vi "sign.vi"() -> ()   [LabVIEW 2020]
uses:
  <vilib>/Utility/file.llb/Read Delimited Spreadsheet (string).vi
  <vilib>/Utility/file.llb/Write Delimited Spreadsheet (string).vi
panel:
  out "output array":string[][](array[string])
  in  "请输入账号":string caption="Please enter your account:"
  in  "请输入密码":string caption="Please enter your password:"
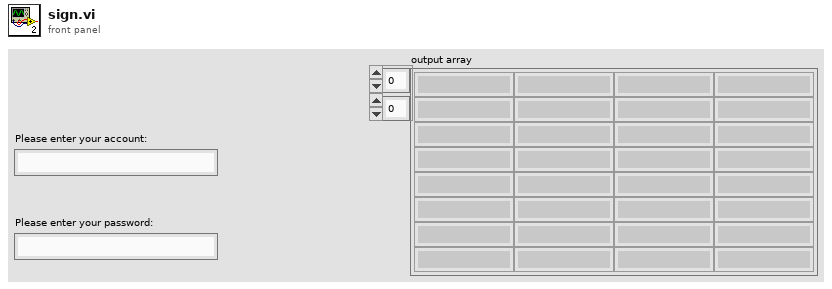
[diagram p1: front panel]
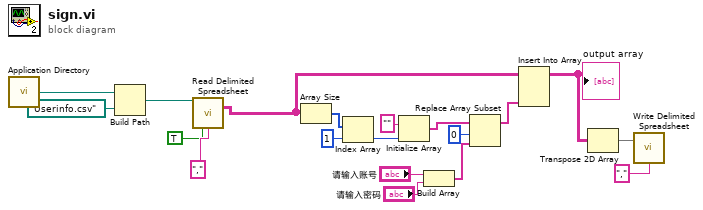
[diagram p0: block diagram]
diagram:
  n1 = call <vilib>:"Application Directory.vi"() -> ("Application Directory"=w19:path)
  n2 = Build Path(base path=w19, name or relative path=path "Userinfo.csv") -> (appended path=w15:path)
  n3 = call-poly <vilib>:"Read Delimited Spreadsheet.vi"("file path (dialog if empty)"=w15, "transpose? (F)"=TRUE, "delimiter (\\t)"="," ("delimiter (\\t)")) -> ("all rows"=w14:string[][])  [unwired: 7 in, 5 out]
  n4 = Array Size(array=w14) -> (size(s)=w11:i32[])
  n5 = Index Array(array=w11, index=1) -> (element=w9:i32)
  n6 = Initialize Array("", w9) -> (w7:string[])
  n7 = Build Array("请输入账号", "请输入密码") -> (w6:string[])
  n8 = Replace Array Subset(array=w7, new element=w6, index=0) -> (w4:string[])
  n9 = Insert Into Array(array=w14, new element=w4) -> (w2:string[][])  [unwired: 2 in]
  "output array" <- w2
  n10 = Transpose 2D Array(2D array=w2) -> (transposed array=w1:string[][])
  n11 = call-poly <vilib>:"Write Delimited Spreadsheet.vi"("2D data"=w1, "delimiter (\\t)"="," ("delimiter (\\t)")) -> ()  [unwired: 12 in, 2 out]
